vi "set default FPS.vi"(8 "error in (no error)":errorcluster, 11 "Thorcam in":refnum<class "Thorcam.lvclass">) -> (0 "error out":errorcluster, 3 "Thorcam out":refnum<class "Thorcam.lvclass">)   [LabVIEW 2012, in "Thorcam.lvclass"]
uses:
  Thorcam.lvclass
  Thorcam.lvclass/Thorcam.ctl
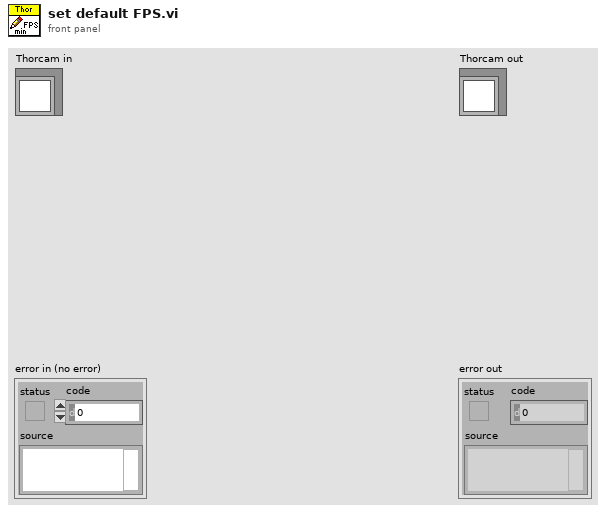
[diagram p1: front panel]
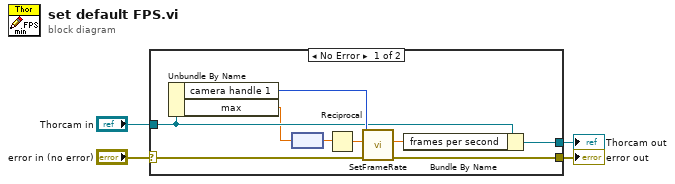
[diagram p0: block diagram]
diagram:
  n1 = case shown="No Error" "error in (no error)" {
    selector: "error in (no error)" -> [w12 w15]
    tunnel: [w11 w15] -> w3
    tunnel: [w9 w14] -> w1
    tunnel: "Thorcam in" -> [w10 w14]
    frame No Error {
      n2 = Unbundle By Name(w10) -> ("camera handle 1"=w13:u32, "max"=w5:dbl[unit])
      n3 = node(w5) -> (w6:dbl)
      n4 = Reciprocal(x=w6) -> (1/x=w7:dbl)
      n5 = call <instrlib>:"SetFrameRate.vi"("error in"=w12, "FPS"=w7, "Camera Handle In"=w13) -> ("error out"=w11:errorcluster, "new FPS"=w8:dbl)  [unwired: 6 in, 1 out]
      n6 = Bundle By Name(cluster=w10, "frames per second"=w8) -> (w9:refnum<class "Thorcam.lvclass">)
    }
    frame Error {
    }
  }
  "error out" <- w3
  "Thorcam out" <- w1
